vi "Read File path.vi"(8 "error in (no error)":errorcluster, 11 "CoSy Config File in":refnum<class "CoSy Config File.lvclass">) -> (0 "error out":errorcluster, 2 "File path":path, 3 "CoSy Config File out":refnum<class "CoSy Config File.lvclass">)   [LabVIEW 2011, in "COSYLib.lvlib" / "CoSy Config File.lvclass"]
uses:
  CoSy Config File.lvclass
  CoSy Config File.lvclass/CoSy Config File.ctl
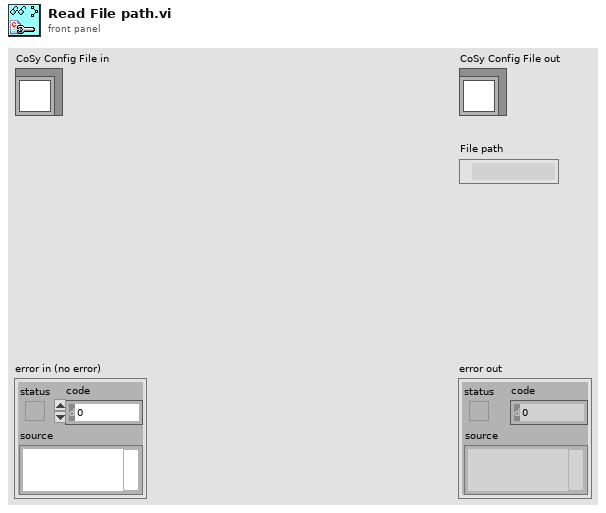
[diagram p1: front panel]
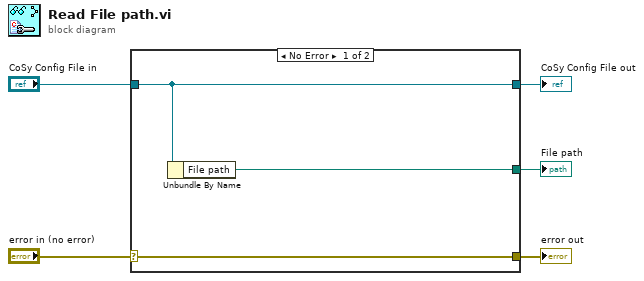
[diagram p0: block diagram]
diagram:
  n1 = case shown="No Error" "error in (no error)" {
    selector: "error in (no error)" -> [w8 w9]
    tunnel: [w8 w9] -> w4
    tunnel: [w7 w10] -> w2
    tunnel: "CoSy Config File in" -> [w7 w10]
    tunnel: [w6 _] -> w1
    frame No Error {
      n2 = Unbundle By Name(w7) -> ("File path"=w6:path)
    }
    frame Error {
    }
  }
  "error out" <- w4
  "CoSy Config File out" <- w2
  "File path" <- w1
